vi "Dashboard Main.vi"() -> ()   [LabVIEW 2016]
uses:
  <vilib>/Utility/miscctls.llb/LVRowAndColumnTypeDef.ctl
  <vilib>/event_ctls.llb/eventvkey.ctl
  <vilib>/Rock Robotics/Network Tables/NT Read Numeric Array.vi
  <vilib>/Rock Robotics/Network Tables/NT Write Numeric Array.vi
  <vilib>/Rock Robotics/Network Tables/NT Write Boolean.vi
  <vilib>/Rock Robotics/WPI/Dashboard/WPI_DashboardLogging Global.vi
panel:
  in  "Camera Settings Right":T1={"Frame Rate"=30, "Compression"=30, "Size"=1, "DB Camera Config"=FALSE} {"Frame Rate" scale=1.0..30.0; "Compression" scale=100.0..-1.0; "Size" items=["640x480", "320x240", "160x120"]}
  in  "Camera Name Right":string(combo)="No Camera Selection"
  out "Camera Info":cluster{"Mbps LED":bool, "Mbps":dbl, "fps":dbl} {"fps" format="%#.1g"; "Mbps" format="%#.1g"}
  in  "Camera Settings":T1={"Frame Rate"=30, "Compression"=30, "Size"=1, "DB Camera Config"=FALSE} {"Frame Rate" scale=1.0..30.0; "Compression" scale=100.0..-1.0; "Size" items=["640x480", "320x240", "160x120"]}
  in  "TCP":refnum<k5>
  in  "Rec Mode":enum32{"Stop", "Record", "Playback"}(radio)
  out "Robot IP":string
  out "Image Message":string="Timeout in Camera Communications"
  in  "Dashboard Tab":T2(tab)
  in  "Robot Centric?":bool
  in  "Scooter Button":bool
  in  "Scooter Scale":dbl(slide)=0.49999999999999994 scale=0.0..1.0
  in  "Select Auto":string(combo)="Select Autonomous ..."
  out "NT Connection":bool
  out "MotorChart R":cluster{"Numeric":dbl, "Numeric":dbl}(graph)
  out "MotorChart L":cluster{"Numeric":dbl, "Numeric":dbl}(graph)
  out "MotorSliders R":cluster{"MotorSlide1":dbl, "MotorSlide2":dbl} {"MotorSlide2" scale=-1.0..1.0 scale format="%#_2e"; "MotorSlide1" scale=-1.0..1.0 scale format="%#_2e"}
  out "MotorSliders L":cluster{"MotorSlide1":dbl, "MotorSlide2":dbl} {"MotorSlide2" scale=-1.0..1.0 scale format="%#_2e"; "MotorSlide1" scale=-1.0..1.0 scale format="%#_2e"}
  out "Gyro":dbl(knob) scale=0.0..360.0
  out "JS1 Z":dbl(slide) scale=-1.0..1.0 scale format="%#_2e"
  out "JS1 Graph":cluster{"X":dbl, "Y":dbl}[](graph)
  out "JS1 Buttons":T3
  out "JS2 Z":dbl(slide) scale=-1.0..1.0 scale format="%#_2e"
  out "JS2 Graph":cluster{"X":dbl, "Y":dbl}[](graph)
  out "JS2 Buttons":T3
  out "Mode":T4(ring)=enum."Auto Disabled"
  out "Camera Image Right":T5(plugin-control)
  in  "DB/String 9":string
  in  "DB/String 8":string
  in  "DB/String 7":string
  in  "DB/String 6":string
  in  "DB/String 5":string
  in  "DB/String 4":string
  in  "DB/String 3":string
  in  "DB/String 2":string
  in  "DB/String 1":string
  in  "DB/String 0":string
  in  "DB/Slider 0":dbl(slide) scale=0.0..5.0
  in  "DB/Slider 1":dbl(slide) scale=0.0..5.0
  in  "DB/Slider 2":dbl(slide) scale=0.0..5.0
  in  "DB/Slider 3":dbl(slide) scale=0.0..5.0
  out "DB/LED 3":bool
  out "DB/LED 2":bool
  out "DB/LED 1":bool
  out "DB/LED 0":bool
  in  "DB/Button 3":bool
  in  "DB/Button 2":bool
  in  "DB/Button 1":bool
  in  "DB/Button 0":bool caption="New Name"
  out "Ultrasonic Distance":dbl
  out "Motor Outputs":T6 {"Motor 7" scale=-1.0..1.0; "Motor 6" scale=-1.0..1.0; "Motor 5" scale=-1.0..1.0; "Motor 4" scale=-1.0..1.0; "Motor 3" scale=-1.0..1.0; "Motor 2" scale=-1.0..1.0; "Motor 1" scale=-1.0..1.0; "Motor 0" scale=-1.0..1.0}
  in  "PID Adjustments":cluster{"P":dbl, "I":dbl, "D":dbl}={"P"=0.3, "I"=0.0, "D"=0.004} {"D" min=0.0 max=10.0 step=0.01; "I" min=0.0 max=10.0 step=0.01; "P" min=0.0 max=10.0 step=0.01}
  out "Encoder Data":dbl[](array[numeric])
  out "NavX Data":dbl[](array[numeric])
  in  "Encoder Offsets":dbl[](array[numeric])
  in  "Test Slider":dbl(slide) scale=0.0..100.0 scale format="%#_3g"
  in  "On/Off":bool caption="Solenoid"
  in  "Test Name":u16(ring) items=["Select the test to run..."]
  in  "Test Tree":string(tree)
  in  "Motor":cluster{"Value":dbl, "Enable":bool} {"Value" scale=-1.0..1.0 scale format="%#_3g"}
  out "Progress":T7 {"Test Progress" scale=0.0..100.0}
  in  "Rev/Fwd":cluster{"Forward":bool, "Reverse":bool}
  in  "Test Ring":u16(ring) items=["Monochrome", "Color"]
  out "Cmd Status":string
  in  "Execute Command":bool
  in  "Command Params":string[][](table)
  in  "Command Selection":i32(listbox)
  in  "CheckList":i32(listbox)
  out "Tree":string(tree)
  out "30 Amp Plugs":dbl[](array[slide]) scale=0.0..30.0
  out "40 Amp Plugs":dbl[](array[slide]) scale=0.0..40.0
  out "Camera Image":T5(plugin-control)
  out "Background":bool
  in  "Camera Name":string(combo)="No Camera Selection"
  # "HW"
  # "HW"
  # "Joysticks"
  # "Drive Motors"
  # "Front"
  # "Right"
  # "Left"
  # "Back"
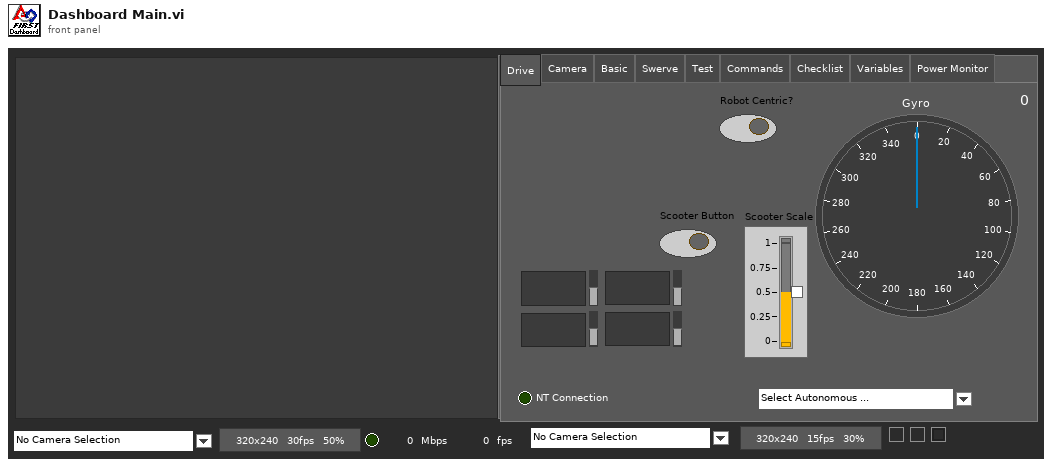
[diagram p1: front panel]
types:
  T1 = cluster{"Frame Rate":i32, "Compression":i32, "Size":u16, "DB Camera Config":bool}
  T2 = enum32{"Drive", "Camera", "Basic", "Swerve", "Test", "Commands", "Checklist", "Variables", "Power Monitor"}
  T3 = cluster{bool, bool, bool, bool, bool, bool, bool, bool, bool, bool, bool, bool}
  T4 = enum8{"Tele-Op Disabled", "Tele-Op Enabled", "Auto Disabled", "Auto Enabled", "Test Disabled", "Test Enabled", "Disconnected", "No Code", "E-Stop"}
  T5 = typedef "IMAQ Image.ctl" = refnum<image>
  T6 = cluster{"Motor 0":dbl, "Motor 1":dbl, "Motor 2":dbl, "Motor 3":dbl, "Motor 4":dbl, "Motor 5":dbl, "Motor 6":dbl, "Motor 7":dbl}
  T7 = cluster{"Test Progress":u8, "Test Progress Text":string}
  T8 = typedef "Image Type" = u32
  T9 = cluster{"IDs":cluster{"RPC field ID":u16, "Unique ID":u16}, "String":string}
  T10 = enum32{"Drive", "Basic", "Custom", "Test", "Checklist", "Variables"}
  T11 = cluster{"Error Strings":string, "Disable Counts":cluster{u16, u16}, "Rail Faults":cluster{u16, u16, u16}, "Robot IP":string, "DB Mode":u8, "Event Info":cluster{"Name":string, "Type":u8, "Number":u16, "Replay":u8}}
  T12 = cluster{"Storage":cluster{"Disk Free":u64, "RAM Block":u32, "RAM free":u32}, "CPU Utilization":cluster{"CPU % ISR":sgl, "CPU % Time Crit":sgl, "CPU % Timed Str":sgl, "CPU % High":sgl, "CPU % Above":sgl, "CPU % Normal":sgl, "CPU % Low":sgl}, "CAN":cluster{"% Bus Utilization":sgl, "Bus Off Cnt":u32, "TX_FIFO Full Cnt":u32, "Receive Error Cnt":u8, "Transmit Error Cnt":u8}, "HID":cluster{"HID Outputs":u32, "Rumble Low":u16, "Rumble High":u16}[]}
  T13 = cluster{"Status bits":cluster{"Test Mode":bool, "Autonomous":bool, "Enabled":bool, "Code Start":bool, "Brownout":bool, "Reserved 2":bool, "Reserved 3":bool, "E-Stop":bool}, "Code Trace":cluster{"Disabled":bool, "TeleOp":bool, "Auto":bool, "Test":bool}, "Controller Type":enum16{"unknown", "cRIO", "roboRio"}, "Code?":enum16{"unknown", "noCode", "code"}, "Battery V":dbl}
  T14 = cluster{"Control Bits":cluster{"TestMode":bool, "Autonomous":bool, "Enabled":bool, "FMS Present":bool, bool, bool, bool, "E-Stop":bool}, "Team Station ":u8, "Countdown":sgl, "Joystick Values":cluster{"Axes":dbl[], "Buttons":bool[], "POVs":i16[]}[]}
  T15 = cluster{"Axes":dbl[], "Buttons":bool[], "POVs":i16[]}[]
  T16 = cluster{"Numeric Array[0]":dbl, "Numeric Array[1]":dbl, "Numeric Array[2]":dbl, "Numeric Array[3]":dbl, "Numeric Array[4]":dbl, "Numeric Array[5]":dbl, "Numeric Array[6]":dbl, "Numeric Array[7]":dbl, "Numeric Array[8]":dbl}
  T17 = cluster{"Numeric Array[0]":dbl, "Numeric Array[1]":dbl, "Numeric Array[2]":dbl, "Numeric Array[3]":dbl, "Numeric Array[4]":dbl, "Numeric Array[5]":dbl, "Numeric Array[6]":dbl, "Numeric Array[7]":dbl}
  T18 = cluster{"Axes":dbl[], "Buttons":bool[], "POVs":i16[]}
  T19 = cluster{"Buttons[0]":bool, "Buttons[1]":bool, "Buttons[2]":bool, "Buttons[3]":bool, "Buttons[4]":bool, "Buttons[5]":bool, "Buttons[6]":bool, "Buttons[7]":bool, "Buttons[8]":bool, "Buttons[9]":bool, "Buttons[10]":bool, "Buttons[11]":bool}
  T20 = cluster{"Camera Image":refnum<vi>, "Dashboard Tab":refnum<vi>, "Background":refnum<vi>, "Rec Mode":refnum<vi>, "Test Slider":refnum<vi>, "On/Off ":refnum<vi>, "Test Ring":refnum<vi>, "Rev/Fwd":refnum<vi>, "Test Name":refnum<vi>, "Motor":refnum<vi>, "Progress":refnum<vi>, "CheckList":refnum<vi>, "Tree":refnum<vi>, "Test Tree":refnum<vi>, "Command Params":refnum<vi>, "Command Selection":refnum<vi>, "Execute Command":refnum<vi>, "Cmd Status":refnum<vi>, "Camera Settings":refnum<vi>, "Camera Name":refnum<vi>, "Camera Info":refnum<vi>, "Camera Settings Right":refnum<vi>, "Camera Name Right":refnum<vi>, "Camera Image Right":refnum<vi>}
  T21 = cluster{"Operation":enum16{"Update", "Clear"}, "Color Box":u32}[]
  T22 = typedef "eventvkey.ctl" = enum16{"ASCII", "Enter", "Return", "Shift", "Ctrl", "Alt", "Cmd", "Opt", "Caps", "NumLock", "Clear", "Break", "Up", "Down", "Left", "Right", "Insert", "Delete", "Home", "End", "PageUp", "PageDown", "Escape", "Help", "Pause", "ScrollLock", "F1", "F2", "F3", "F4", "F5", "F6", "F7", "F8", "F9", "F10", "F11", "F12", "F13", "F14", "F15", "F16", "F17", "F18", "F19", "F20", "F21", "F22", "F23", "F24", "Play", "VolumeUp", "VolumeDown", "Mute", "Two Byte Char"}
  T23 = cluster{"Image Size":bool, "Image Type":bool, "Pixel Value":bool, "ROI Information":bool, "Zoom Factor":bool}
  T24 = cluster{"Operation":enum16{"Update", "Clear"}, "Color Box":u32}
  T25 = typedef "LVRowAndColumnTypeDef.ctl" = cluster{"Row":i32, "Column":i32}
  T26 = cluster{"Shift":bool, "Ctrl":bool, "Alt":bool, "Cmd":bool, "Opt":bool}
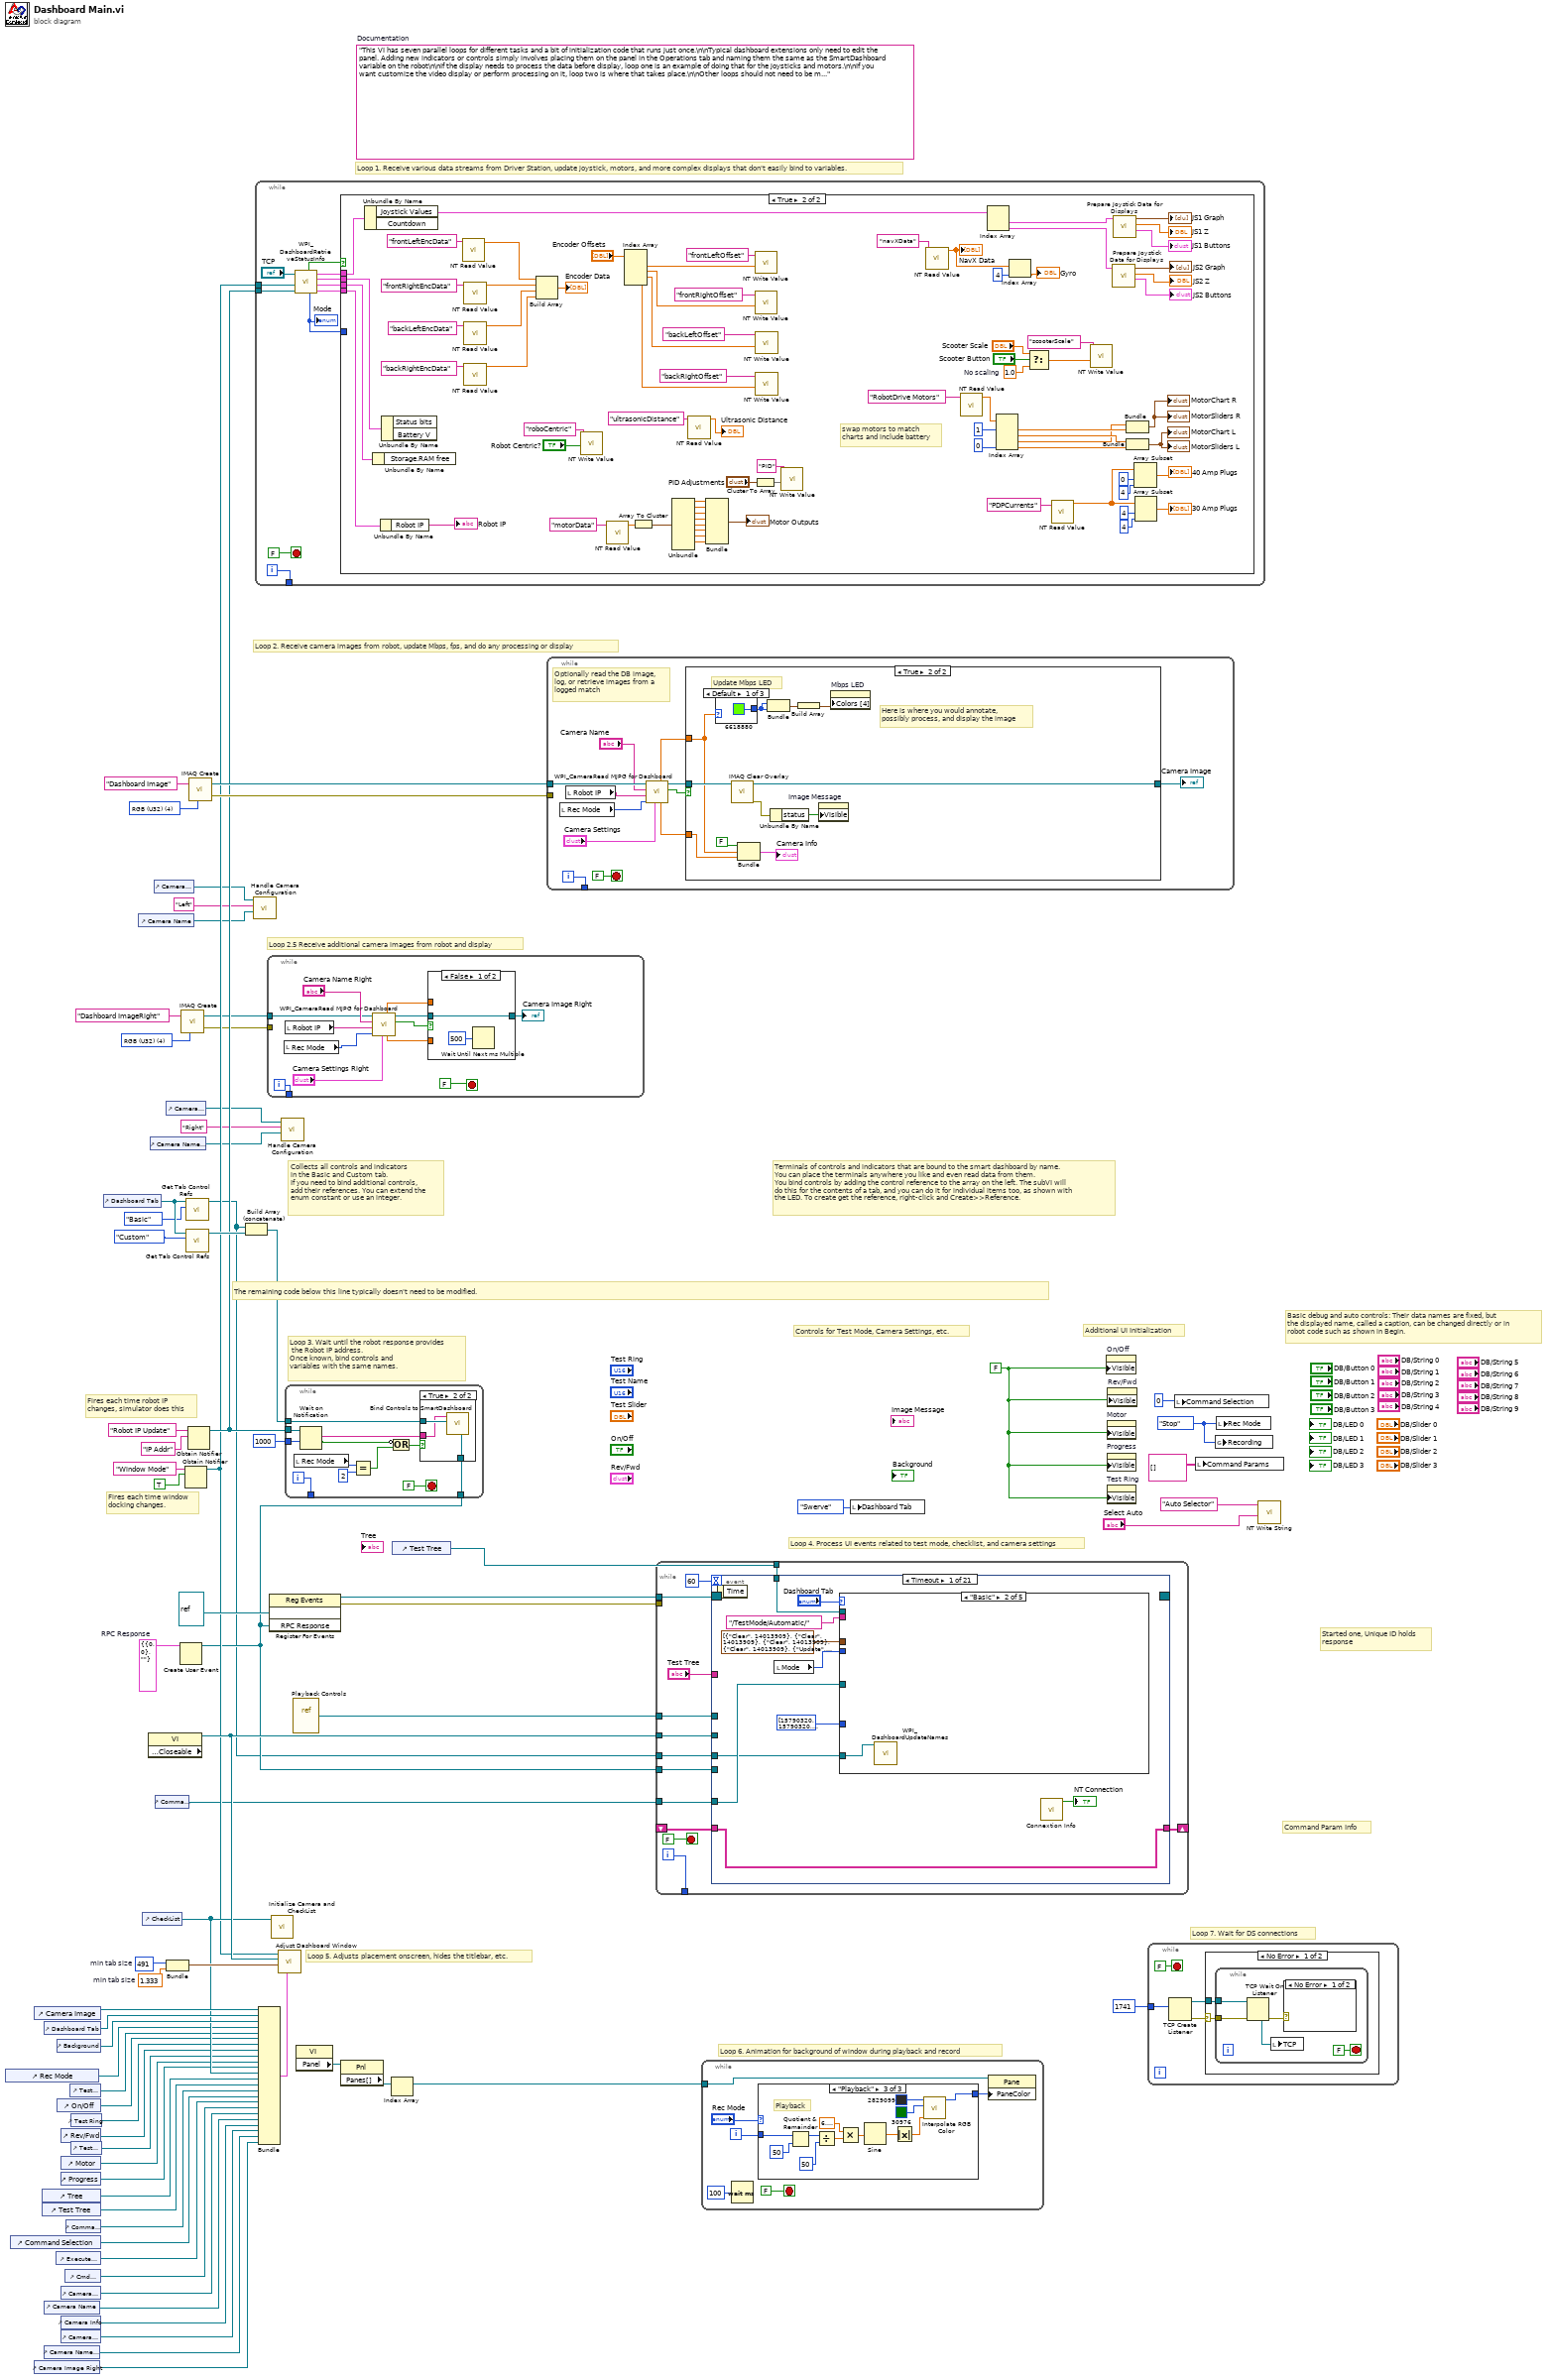
[diagram p0: block diagram]
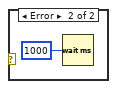
[diagram p3: hidden frame]
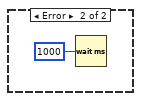
[diagram p4: hidden frame]
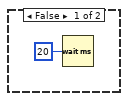
[diagram p5: hidden frame]
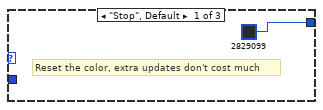
[diagram p6: hidden frame]
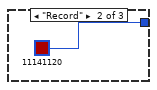
[diagram p7: hidden frame]
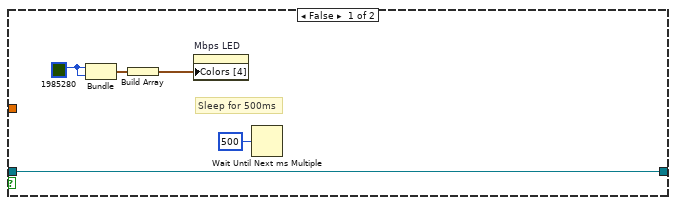
[diagram p9: hidden frame]
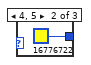
[diagram p10: hidden frame]
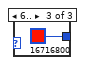
[diagram p11: hidden frame]
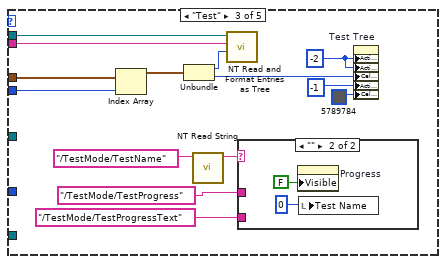
[diagram p13: hidden frame]
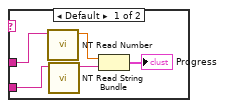
[diagram p14: hidden frame]
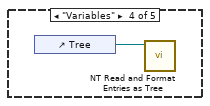
[diagram p15: hidden frame]
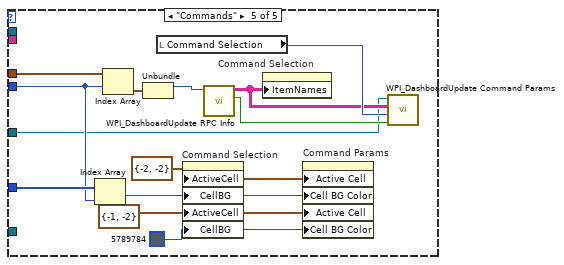
[diagram p16: hidden frame]
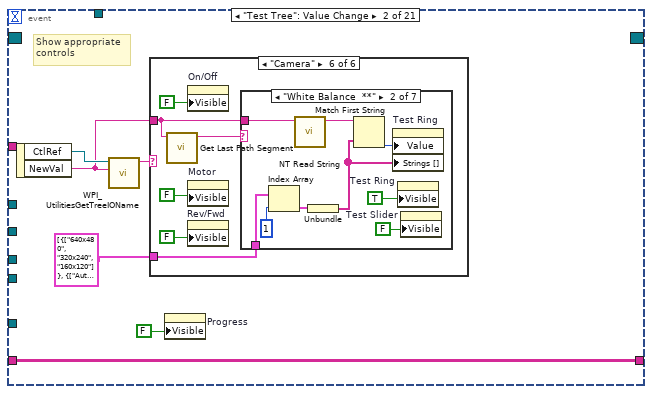
[diagram p17: hidden frame]
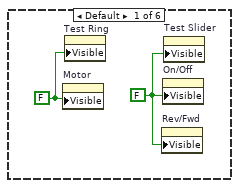
[diagram p18: hidden frame]
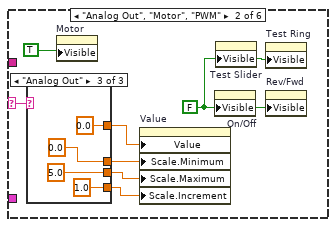
[diagram p19: hidden frame]
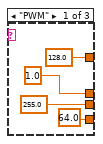
[diagram p20: hidden frame]
diagram:
  w11 = T8 4 items=["Grayscale (U8)", "Grayscale (I16)", "Grayscale (SGL)", "Complex (CSG)", "RGB (U32)", "HSL (U32)", "RGB (U64)"] ("Image Type")
  w27 = T9 {"IDs"={"RPC field ID"=0, "Unique ID"=0}, "String"=""}  # RPC Response
  w51 = 491  # min tab size
  w50 = 1.333  # min tab size
  w58 = enum32{"Stop", "Record", "Playback"}."Stop" ("Rec Mode")
  w33 = FALSE ("Visible")
  (unwired) "This VI has seven parallel loops for different tasks and a bit of initialization code that runs just once.\n\nTypical dashboard extensions only need to edit the panel. Adding new indicators or controls simply involves placing them on the panel in the Operations tab and naming them the same as the SmartDashboard variable on the robot\n\nIf the display needs to process the data before display, loop one is an example of doing that for the joysticks and motors.\n\nIf you want customize the video display or perform processing on it, loop two is where that takes place.\n\nOther loops should not need to be modified. They are pretty standard, and document the task they perform."  # Documentation
  w75 = T8 4 items=["Grayscale (U8)", "Grayscale (I16)", "Grayscale (SGL)", "Complex (CSG)", "RGB (U32)", "HSL (U32)", "RGB (U64)"] ("Image Type")
  # "Loop 2.5 Receive additional camera images from robot and display"
  # "Command Param Info"
  # "Started one, Unique ID holds\nresponse"
  # "Loop 7. Wait for DS connections"
  # "Basic debug and auto controls: Their data names are fixed, but\nthe displayed name, called a caption, can be changed directly or in\nrobot code such as shown in Begin."
  # "Controls for Test Mode, Camera Settings, etc."
  # "Additional UI Initialization"
  # "Loop 6. Animation for background of window during playback and record"
  # "Fires each time robot IP\nchanges, simulator does this"
  # "Fires each time window\ndocking changes."
  # "Collects all controls and indicators\nin the Basic and Custom tab.\nIf you need to bind additional controls,\nadd their references. You can extend the\nenum constant or use an integer."
  # "The remaining code below this line typically doesn't need to be modified."
  # "Loop 4. Process UI events related to test mode, checklist, and camera settings"
  # "Terminals of controls and indicators that are bound to the smart dashboard by name.\nYou can place the terminals anywhere you like and even read data from them.\nYou bind controls by adding the control reference to the array on the left. The subVI will\ndo this for the contents of a tab, and you can do it for individual items too, as shown with\nthe LED. To create get the reference, right-click and Create>>Reference."
  # "Loop 3. Wait until the robot response provides\n the Robot IP address.\nOnce known, bind controls and\nvariables with the same names."
  # "Loop 5. Adjusts placement onscreen, hides the titlebar, etc."
  # "Loop 1. Receive various data streams from Driver Station, update joystick, motors, and more complex displays that don't easily bind to variables."
  # "Loop 2. Receive camera images from robot, update Mbps, fps, and do any processing or display"
  n1 = control-ref of="Rec Mode"() -> (w39:refnum<vi>)
  n2 = control-ref of="Command Selection"() -> (w26:refnum<vi>)
  n3 = control-ref of="Camera Image Right"() -> (w2:refnum<vi>)
  n4 = control-ref of="Camera Image"() -> (w53:refnum<vi>)
  n5 = control-ref of="Tree"() -> (w43:refnum<vi>)
  n6 = control-ref of="Test Tree"() -> (w42:refnum<vi>)
  n7 = control-ref of="Dashboard Tab"() -> (w52:refnum<vi>)
  n8 = control-ref of="Camera Name"() -> (w17:refnum<vi>)
  n9 = control-ref of="Camera Name Right"() -> (w3:refnum<vi>)
  n10 = control-ref of="Execute Command"() -> (w28:refnum<vi>)
  n11 = control-ref of="Background"() -> (w48:refnum<vi>)
  n12 = control-ref of="On/Off"() -> (w37:refnum<vi>)
  n13 = control-ref of="Progress"() -> (w34:refnum<vi>)
  n14 = control-ref of="Camera Settings"() -> (w18:refnum<vi>)
  n15 = control-ref of="Camera Info"() -> (w16:refnum<vi>)
  n16 = control-ref of="Camera Settings Right"() -> (w4:refnum<vi>)
  n17 = control-ref of="Rev/Fwd"() -> (w35:refnum<vi>)
  n18 = control-ref of="Motor"() -> (w40:refnum<vi>)
  n19 = control-ref of="Cmd Status"() -> (w22:refnum<vi>)
  n20 = control-ref of="Command Params"() -> (w29:refnum<vi>)
  n21 = control-ref of="Test Slider"() -> (w38:refnum<vi>)
  n22 = control-ref of="Test Ring"() -> (w36:refnum<vi>)
  n23 = control-ref of="Test Name"() -> (w41:refnum<vi>)
  n24 = control-ref of="Dashboard Tab"() -> (w56:refnum<vi>)
  n25 = control-ref of="Camera Name"() -> (w19:refnum<vi>)
  n26 = control-ref of="CheckList"() -> (w44:refnum<vi>)
  n27 = property class="VI" props=["Front Panel.Closeable"]() -> (reference out=w57:refnum<vi>)  [unwired: 2 in, 2 out]
  n28 = control-ref of="Camera Name Right"() -> (w7:refnum<vi>)
  n29 = control-ref of="Camera Settings"() -> (w20:refnum<vi>)
  n30 = control-ref of="Command Params"() -> (w21:refnum<vi>)
  n31 = control-ref of="Camera Settings Right"() -> (w8:refnum<vi>)
  n32 = Bundle("min tab size"=w51, "min tab size"=w50) -> (w49:cluster{"min tab size":i32, "min tab size":dbl})  [unwired: 1 in]
  n33 = Create User Event(user event datatype=w27) -> (user event=w23:refnum<user-event>)  [unwired: 1 in, 1 out]
  n34 = call "IMAQ Create"("Image Name"="Dashboard ImageRight", "Image Type"=w11) -> ("New Image"=w10:T5, "error out"=w9:errorcluster)  [unwired: 2 in, 1 out]
  n35 = Obtain Notifier(name (unnamed)="Window Mode", notification data type=TRUE) -> (notifier out=w31:refnum<notifier>)  [unwired: 2 in, 2 out]
  n36 = call <vilib>:"Get Tab Control Refs.vi"("Page Index"=T10."Basic" ("Dashboard Tab"), "TabControl in"=w56) -> ("ControlsOnPage"=w15:refnum<vi>[])  [unwired: 9 in]
  n37 = call <vilib>:"Get Tab Control Refs.vi"("Page Index"=T10."Custom" ("Dashboard Tab"), "TabControl in"=w56) -> ("ControlsOnPage"=w55:refnum<vi>[])  [unwired: 9 in]
  n38 = Obtain Notifier(name (unnamed)="Robot IP Update", notification data type="IP Addr" ("name (unnamed)")) -> (notifier out=w32:refnum<notifier>)  [unwired: 2 in, 2 out]
  n39 = call "IMAQ Create"("Image Name"="Dashboard Image", "Image Type"=w75) -> ("New Image"=w73:T5, "error out"=w72:errorcluster)  [unwired: 2 in, 1 out]
  n40 = Build Array (concatenate)(w15, w55) -> (w54:refnum<vi>[])
  n41 = call "Handle Camera Configuration.vi"("CameraNameRef"=w19, "Camera File Name"="Left", "ClusterRef"=w20) -> ()  [unwired: 9 in]
  n42 = while {
    tunnel: [w85] -> _
    tunnel: w32 -> [w79]
    tunnel: w31 -> [w76]
    i -> [w85]
    stop <- FALSE stop-if-true
    n43 = call <vilib>:"WPI_DashboardRetrieveStatusInfo.vi"("Binding Refnum"=w79, "Window Mode Notifier"=w76, "TCP Cnx"="TCP") -> ("Power and Errors"=w80:T11, "Robot Metrics"=w83:T12, "Status Info"=w84:T13, "Control Info"=w81:T14, "Robot Mode"=w78:T4, "Process?"=w82:bool)  [unwired: 3 in]
    "Mode" <- w78
    n44 = case shown="True" w82 {
      tunnel: w84 -> [_ w165]
      tunnel: w83 -> [_ w164]
      tunnel: w81 -> [_ w163]
      tunnel: w80 -> [_ w162]
      tunnel: w78 -> [_ _]
      frame False {
        n45 = Wait (ms)(milliseconds to wait=u32 20) -> ()  [unwired: 1 out]
      }
      frame True {
        w94 = 1.0  # No scaling
        # "swap motors to match\ncharts and include battery"
        n46 = Unbundle By Name(w163) -> ("Joystick Values"=w153:T15)  [unwired: 1 out]
        n47 = Unbundle By Name(w164) -> ()  [unwired: 1 out]
        n48 = Unbundle By Name(w162) -> ("Robot IP"=→"Robot IP":string)
        n49 = Unbundle By Name(w165) -> ()  [unwired: 2 out]
        n50 = call-poly <vilib>:"NT Read Value.vi"("Name"="frontLeftEncData") -> ("Numeric"=w127:dbl)  [unwired: 9 in, 1 out]
        n51 = call-poly <vilib>:"NT Read Value.vi"("Name"="frontRightEncData") -> ("Numeric"=w126:dbl)  [unwired: 9 in, 1 out]
        n52 = call-poly <vilib>:"NT Read Value.vi"("Name"="backLeftEncData") -> ("Numeric"=w125:dbl)  [unwired: 9 in, 1 out]
        n53 = call-poly <vilib>:"NT Read Value.vi"("Name"="backRightEncData") -> ("Numeric"=w124:dbl)  [unwired: 9 in, 1 out]
        n54 = Build Array(w127, w126, w125, w124) -> (→"Encoder Data":dbl[])
        n55 = call-poly <vilib>:"NT Write Value.vi"("Boolean"="Robot Centric?", "Name"="roboCentric") -> ()  [unwired: 9 in, 1 out]
        n56 = call-poly <vilib>:"NT Read Value.vi"("Name"="motorData") -> ("Numeric Array"=w118:dbl[])  [unwired: 9 in, 1 out]
        n57 = Index Array(array="Encoder Offsets") -> (element #1=w135:dbl, element #2=w134:dbl, element #3=w133:dbl, element #4=w132:dbl)  [unwired: 4 in]
        n58 = Array To Cluster(array=w118) -> (cluster=w117:T16)
        n59 = Unbundle(w117) -> ("Numeric Array[0]"=w116:dbl, "Numeric Array[1]"=w115:dbl, "Numeric Array[2]"=w114:dbl, "Numeric Array[3]"=w113:dbl, "Numeric Array[4]"=w112:dbl, "Numeric Array[5]"=w111:dbl, "Numeric Array[6]"=w110:dbl, "Numeric Array[7]"=w109:dbl)  [unwired: 1 out]
        n60 = call-poly <vilib>:"NT Read Value.vi"("Name"="ultrasonicDistance") -> ("Numeric"=→"Ultrasonic Distance":dbl)  [unwired: 9 in, 1 out]
        n61 = Bundle("Numeric Array[0]"=w116, "Numeric Array[1]"=w115, "Numeric Array[2]"=w114, "Numeric Array[3]"=w113, "Numeric Array[4]"=w112, "Numeric Array[5]"=w111, "Numeric Array[6]"=w110, "Numeric Array[7]"=w109) -> (→"Motor Outputs":T17)  [unwired: 1 in]
        n62 = Cluster To Array(cluster="PID Adjustments") -> (array=w121:dbl[])
        n63 = call-poly <vilib>:"NT Write Value.vi"("Numeric"=w135, "Name"="frontLeftOffset") -> ()  [unwired: 9 in, 1 out]
        n64 = call-poly <vilib>:"NT Write Value.vi"("Numeric"=w134, "Name"="frontRightOffset") -> ()  [unwired: 9 in, 1 out]
        n65 = call-poly <vilib>:"NT Write Value.vi"("Numeric"=w133, "Name"="backLeftOffset") -> ()  [unwired: 9 in, 1 out]
        n66 = call-poly <vilib>:"NT Write Value.vi"("Numeric"=w132, "Name"="backRightOffset") -> ()  [unwired: 9 in, 1 out]
        n67 = call-poly <vilib>:"NT Write Value.vi"("Numeric Array"=w121, "Name"="PID") -> ()  [unwired: 9 in, 1 out]
        n68 = call-poly <vilib>:"NT Read Value.vi"("Name"="navXData") -> ("Numeric Array"=w107:dbl[])  [unwired: 9 in, 1 out]
        "NavX Data" <- w107
        n69 = call-poly <vilib>:"NT Read Value.vi"("Name"="RobotDrive Motors") -> ("Numeric Array"=w143:dbl[])  [unwired: 9 in, 1 out]
        n70 = Index Array(array=w153) -> (element #1=w152:T18, element #2=w148:T18)  [unwired: 2 in]
        n71 = Index Array(array=w143, index #1=1, index #4=0) -> (element #1=w157:dbl, element #2=w158:dbl, element #3=w156:dbl, element #4=w161:dbl)  [unwired: 2 in]
        n72 = Index Array(array=w107, index=4) -> (element=→"Gyro":dbl)
        n73 = Select(t="Scooter Scale", s="Scooter Button", f=w94) -> (s? t:f=w93:dbl)
        n74 = call-poly <vilib>:"NT Read Value.vi"("Name"="PDPCurrents") -> ("Numeric Array"=w101:dbl[])  [unwired: 9 in, 1 out]
        n75 = call-poly <vilib>:"NT Write Value.vi"("Numeric"=w93, "Name"="scooterScale") -> ()  [unwired: 9 in, 1 out]
        n76 = call "Prepare Joystick Data for Displays.vi"("Joystick Values"=w148) -> ("Buttons"=→"JS2 Buttons":T19, "Z Axis"=→"JS2 Z":dbl, "Cartesian Data"=→"JS2 Graph":cluster{"X axis":dbl, "X axis":dbl}[])  [unwired: 8 in]
        n77 = call "Prepare Joystick Data for Displays.vi"("Joystick Values"=w152) -> ("Buttons"=→"JS1 Buttons":T19, "Z Axis"=→"JS1 Z":dbl, "Cartesian Data"=→"JS1 Graph":cluster{"X axis":dbl, "X axis":dbl}[])  [unwired: 8 in]
        n78 = Bundle("Numeric"=w156, "Numeric"=w157) -> (→"MotorChart R" →"MotorSliders R":cluster{"Numeric":dbl, "Numeric":dbl})  [unwired: 1 in]
        n79 = Bundle("Numeric"=w158, "Numeric"=w161) -> (→"MotorChart L" →"MotorSliders L":cluster{"Numeric":dbl, "Numeric":dbl})  [unwired: 1 in]
        n80 = Array Subset(array=w101, index=0, length=4) -> (→"40 Amp Plugs":dbl[])
        n81 = Array Subset(array=w101, index=4, length=4) -> (→"30 Amp Plugs":dbl[])
      }
    }
  }
  n82 = Bundle("Camera Image"=w53, "Dashboard Tab"=w52, "Background"=w48, "Rec Mode"=w39, "Test Slider"=w38, "On/Off"=w37, "Test Ring"=w36, "Rev/Fwd"=w35, "Test Name"=w41, "Motor"=w40, "Progress"=w34, "CheckList"=w44, "Tree"=w43, "Test Tree"=w42, "Command Params"=w29, "Command Selection"=w26, "Execute Command"=w28, "Cmd Status"=w22, "Camera Settings"=w18, "Camera Name"=w17, "Camera Info"=w16, "Camera Settings Right"=w4, "Camera Name Right"=w3, "Camera Image Right"=w2) -> (w45:T20)  [unwired: 1 in]
  n83 = while {
    tunnel: w10 -> [w176]
    tunnel: w9 -> [_]
    tunnel: [w170] -> _
    i -> [w170]
    stop <- FALSE stop-if-true
    n84 = local read "Rec Mode"() -> (w174:enum32{"Stop", "Record", "Playback"})
    n85 = local read "Robot IP"() -> (w175:string)
    n86 = call <vilib>:"WPI_CameraRead MJPG for Dashboard.vi"("Camera Settings"="Camera Settings Right", "Rec Mode"=w174, "Robot IP"=w175, "Camera Name"="Camera Name Right", "Refnum in"=w176) -> ("Active"=w169:bool, "Refnum out"=w172:T5, "FPS"=w167:dbl, "Bandwidth (Mbps)"=w168:dbl)  [unwired: 3 in]
    n87 = case shown="False" w169 {
      tunnel: w172 -> [w178 w180]
      tunnel: w168 -> [_ _]
      tunnel: w167 -> [_ _]
      tunnel: [w178 w180] -> w166
      frame False {
        n88 = Wait Until Next ms Multiple(millisecond multiple=u32 500) -> ()  [unwired: 1 out]
      }
      frame True {
      }
    }
    "Camera Image Right" <- w166
  }
  n89 = register-events(refnum<vi> refnum, w23) -> (reference out=w62:refnum<event-registration>, error out=w61:errorcluster)  [unwired: 2 in]
  n90 = call "Initialize Camera and CheckList.vi"("ListBox in"=w44) -> ()  [unwired: 11 in]
  n91 = call "Adjust Dashboard Window.vi"("Sizing Refnums"=w45, "Size Constraints"=w49, "VI"=w57, "WIn Mode"=w31) -> ()  [unwired: 8 in]
  n92 = call "Handle Camera Configuration.vi"("CameraNameRef"=w7, "Camera File Name"="Right", "ClusterRef"=w8) -> ()  [unwired: 9 in]
  n93 = while {
    tunnel: w54 -> [w192]
    tunnel: w32 -> [w190]
    tunnel: [w188] -> _
    tunnel: u32 1000 ("milliseconds to wait") -> [w187]
    tunnel: w23 -> [w181]
    i -> [w188]
    stop <- FALSE stop-if-true
    n94 = local read "Rec Mode"() -> (w183:enum32{"Stop", "Record", "Playback"})
    n95 = Wait on Notification(notifier=w190, timeout in ms (-1)=w187) -> (notification=w189:string, timed out?=w185:bool)  [unwired: 2 in, 2 out]
    n96 = Equal?(x=w183, y=u16 2 ("Rec Mode")) -> (x = y?=w184:bool)
    n97 = Compound Arithmetic op=OR(invert w185, w184) -> (w186:bool)
    n98 = case shown="True" w186 {
      tunnel: w192 -> [_ w195]
      tunnel: w189 -> [_ w194]
      tunnel: w181 -> [_ w193]
      frame False {
      }
      frame True {
        n99 = call <vilib>:"Bind Controls to SmartDashboard.vi"("RPC ref"=w193, "Bound Control Refs"=w195, "Server IP Address"=w194) -> ()  [unwired: 9 in]
      }
    }
  }
  n100 = vi-ref "Playback Controls.vi"() -> (w63:refnum<vi>)
  n101 = property class="VI"() -> ("Panel"=w65:refnum<vi>)  [unwired: 2 in, 2 out]
  n102 = property class="Pnl"(reference=w65) -> ("Panes[]"=w66:refnum<vi>[])  [unwired: 1 in, 2 out]
  n103 = Index Array(array=w66) -> (element=w64:refnum<vi>)  [unwired: 1 in]
  n104 = control-ref of="Test Tree"() -> (w67:refnum<vi>)
  n105 = while {
    tunnel: w73 -> [w205]
    tunnel: w72 -> [_]
    tunnel: [w206] -> _
    i -> [w206]
    stop <- FALSE stop-if-true
    # "Optionally read the DB image,\nlog, or retrieve images from a\nlogged match"
    n106 = local read "Rec Mode"() -> (w201:enum32{"Stop", "Record", "Playback"})
    n107 = local read "Robot IP"() -> (w200:string)
    n108 = call <vilib>:"WPI_CameraRead MJPG for Dashboard.vi"("Camera Settings"="Camera Settings", "Rec Mode"=w201, "Robot IP"=w200, "Camera Name"="Camera Name", "Refnum in"=w205) -> ("Active"=w203:bool, "Refnum out"=w204:T5, "FPS"=w202:dbl, "Bandwidth (Mbps)"=w199:dbl)  [unwired: 3 in]
    n109 = case shown="True" w203 {
      tunnel: w204 -> [w208 w219]
      tunnel: w199 -> [_ w216]
      tunnel: w202 -> [_ w217]
      tunnel: [w208 w213] -> w196
      frame False {
        w210 = u32 1985280 ("Color Box")
        # "Sleep for 500ms"
        n110 = Bundle("Color Box"=w210, "Color Box"=w210) -> (w211:cluster{"Color Box":u32, "Color Box":u32})  [unwired: 1 out]
        n111 = Build Array(w211) -> (w209:cluster{"Color Box":u32, "Color Box":u32}[])
        n112 = property on="Mbps LED" class="Bool (strict)"("Colors [4]"=w209) -> ()  [unwired: 2 in, 2 out]
        n113 = Wait Until Next ms Multiple(millisecond multiple=u32 500) -> ()  [unwired: 1 out]
      }
      frame True {
        # "Here is where you would annotate,\npossibly process, and display the image"
        # "Update Mbps LED"
        n114 = case shown="Default" w216 {
          tunnel: [u32 6618880 ("Color Box") u32 16776722 ("Color Box") u32 16716800 ("Color Box")] -> w220
          frame Default {
          }
          frame 4, 5 {
          }
          frame 6.. {
          }
        }
        n115 = call "IMAQ Clear Overlay"("Image"=w219) -> ("error out"=w222:errorcluster, "Image Out"=w213:T5)  [unwired: 2 in, 7 out]
        n116 = Bundle(FALSE, "Bandwidth (Mbps)"=w216, "FPS"=w217) -> (→"Camera Info":cluster{bool, "Bandwidth (Mbps)":dbl, "FPS":dbl})  [unwired: 1 in]
        n117 = Bundle("Color Box"=w220, "Color Box"=w220) -> (w221:cluster{"Color Box":u32, "Color Box":u32})  [unwired: 1 out]
        n118 = Unbundle By Name(w222) -> ("status"=w223:bool)
        n119 = Build Array(w221) -> (w218:cluster{"Color Box":u32, "Color Box":u32}[])
        n120 = property on="Image Message" class="Str"("Visible"=w223) -> ()  [unwired: 2 in, 2 out]
        n121 = property on="Mbps LED" class="Bool (strict)"("Colors [4]"=w218) -> ()  [unwired: 2 in, 2 out]
      }
    }
    "Camera Image" <- w196
  }
  n122 = while {
    tunnel: [w236] -> _
    tunnel: w67 -> [w235]
    tunnel: w63 -> [w234]
    tunnel: w62 -> [w233]
    tunnel: w61 -> [_]
    tunnel: w57 -> [w232]
    tunnel: w23 -> [w231]
    tunnel: w21 -> [w230]
    shift-right: [w229] -> _
    shift-left: _ -> [w228]
    tunnel: w15 -> [w227]
    i -> [w236]
    stop <- FALSE stop-if-true
    n123 = event shown="[0] Timeout" {
      selector: w233 -> [_ _ _ _ _ _ _ _ _ _ _ _ _ _ _ _ _ _ _ _ _]
      dyn-events: [_ _ _ _ _ _ _ _ _ _ _ _ _ _ _ _ w492 _ _ _ _] -> _
      timeout: u32 60 ("milliseconds to wait") -> [_ _ _ _ _ _ _ _ _ _ _ _ _ _ _ _ _ _ _ _ _]
      tunnel: w235 -> [w248 _ _ _ _ _ _ _ _ _ _ _ _ _ _ _ _ _ _ _ _]
      tunnel: "Test Tree" -> [_ _ _ _ _ _ _ _ _ _ _ w459 w467 w469 w473 w481 _ _ _ _ _]
      tunnel: w234 -> [_ _ _ _ _ _ _ _ _ _ _ _ _ _ _ _ w494 _ w512 _ _]
      tunnel: w232 -> [_ _ _ _ _ _ _ _ _ _ _ _ _ _ _ _ w490 _ _ _ _]
      tunnel: w231 -> [_ _ _ _ _ _ _ _ _ _ _ _ _ _ _ _ w486 _ _ _ _]
      tunnel: w230 -> [w243 _ _ _ _ _ w410 _ _ _ _ _ _ _ _ _ _ _ _ _ _]
      tunnel: [w242 w287 w389 w394 w403 w407 w408 w417 w427 w434 w446 w458 w465 w468 w472 w480 w485 w507 w509 w513 w524] -> w229
      tunnel: w228 -> [w242 w287 w389 w394 w403 w407 w408 _ _ w434 w446 w458 w465 w468 w472 w480 w485 w507 w509 w513 w524]
      tunnel: w227 -> [w240 _ _ _ _ _ _ _ _ _ _ _ _ _ _ _ _ _ _ _ _]
      event Timeout {
        n124 = event-data() -> ()  [unwired: 1 in, 1 out]
        n125 = local read "Mode"() -> (w245:T4)
        n126 = case shown="\"Basic\"" "Dashboard Tab" {
          tunnel: w248 -> [_ _ w264 _ _]
          tunnel: "/TestMode/Automatic/" ("Name Pattern") -> [_ _ w263 _ _]
          tunnel: T21 [{"Operation"=enum."Clear", "Color Box"=14013909}, {"Operation"=enum."Clear", "Color Box"=14013909}, {"Operation"=enum."Clear", "Color Box"=14013909}, {"Operation"=enum."Clear", "Color Box"=14013909}, {"Operation"=enum."Update", "Color Box"=14013909}, {"Operation"=enum."Update", "Color Box"=16777215}, {"Operation"=enum."Clear", "Color Box"=14013909}, {"Operation"=enum."Clear", "Color Box"=14013909}, {"Operation"=enum."Clear", "Color Box"=14013909}] -> [_ _ w256 _ w280]
          tunnel: w245 -> [_ _ w255 _ w279]
          tunnel: u32[] [15790320, 15790320, 15790320, 15790320, 16777215, 16777215, 15790320, 15790320, 15790320] -> [_ _ _ _ w285]
          tunnel: w243 -> [_ _ _ _ w273]
          tunnel: w240 -> [_ w250 _ _ _]
          frame "Swerve", Default {
          }
          frame "Basic" {
            n127 = call <vilib>:"WPI_DashboardUpdateNames.vi"("Controls on Tab"=w250) -> ()  [unwired: 11 in]
          }
          frame "Test" {
            w262 = -2 ("Active Item:Row Number")
            n128 = Index Array(array=w256, index=w255) -> (element=w257:T24)
            n129 = Unbundle(w257) -> ("Operation"=w258:enum16{"Update", "Clear"}, "Color Box"=w259:u32)
            n130 = call <vilib>:"NT Read String.vi"("Name"="/TestMode/TestName") -> ("String"=w253:string)  [unwired: 9 in, 1 out]
            n131 = call <vilib>:"NT Read and Format Entries as Tree.vi"("Operation"=w258, "Name Pattern"=w263, "Tree Refnum"=w264) -> ()  [unwired: 7 in, 2 out]
            n132 = case shown="\"\"" w253 {
              tunnel: "/TestMode/TestProgress" ("Name") -> [w266 _]
              tunnel: "/TestMode/TestProgressText" ("Name") -> [w265 _]
              frame Default {
                n133 = call <vilib>:"NT Read Number.vi"("Name"=w266) -> ("Numeric"=w267:dbl)  [unwired: 9 in, 1 out]
                n134 = call <vilib>:"NT Read String.vi"("Name"=w265) -> ("String"=w268:string)  [unwired: 9 in, 1 out]
                n135 = Bundle("Numeric"=w267, "String"=w268) -> (→"Progress":cluster{"Numeric":dbl, "String":string})  [unwired: 1 in]
              }
              frame "" {
                n136 = property on="Progress" class="Clust (strict)"("Visible"=FALSE) -> ()  [unwired: 2 in, 2 out]
                n137 = local write "Test Name"(u16 0) -> ()
              }
            }
            n138 = property on="Test Tree" class="Tree (strict)"("Active Item Row Number"=w262, "ActiveColNum"=w262, "CellBG"=w259, "Active Item Row Number"=-1 ("Active Item:Row Number"), "CellBG"=u32 5789784 ("Color Box")) -> ()  [unwired: 2 in, 2 out]
          }
          frame "Variables" {
            n139 = control-ref of="Tree"() -> (w272:refnum<vi>)
            n140 = call <vilib>:"NT Read and Format Entries as Tree.vi"("Tree Refnum"=w272) -> ()  [unwired: 9 in, 2 out]
          }
          frame "Commands" {
            w281 = u32 5789784 ("Color Box")
            w282 = T25 {"Row"=-1, "Column"=-2} ("Active Cell:Active Cell")
            w284 = T25 {"Row"=-2, "Column"=-2} ("Active Cell:Active Cell")
            n141 = Index Array(array=w285, index=w279) -> (element=w283:u32)
            n142 = Index Array(array=w280, index=w279) -> (element=w278:T24)
            n143 = Unbundle(w278) -> ("Operation"=w277:enum16{"Update", "Clear"})  [unwired: 1 out]
            n144 = local read "Command Selection"() -> (w276:i32)
            n145 = property on="Command Selection" class="MCListbox (strict)"("ActiveCell"=w284, "CellBG"=w283, "ActiveCell"=w282, "CellBG"=w281) -> ()  [unwired: 2 in, 2 out]
            n146 = call <vilib>:"WPI_DashboardUpdate RPC Info.vi"("Operation"=w277) -> ("update"=w275:bool, "commands"=w274:string[][])  [unwired: 9 in]
            n147 = property on="Command Selection" class="MCListbox (strict)"("ItemNames"=w274) -> ()  [unwired: 2 in, 2 out]
            n148 = property on="Command Params" class="Tbl (strict)"("Active Cell"=w284, "Cell BG Color"=w283, "Active Cell"=w282, "Cell BG Color"=w281) -> ()  [unwired: 2 in, 2 out]
            n149 = call <vilib>:"WPI_DashboardUpdate Command Params.vi"("Update"=w275, "NewVal"=w276, "Commands"=w274, "Param Tbl"=w273) -> ()  [unwired: 7 in, 1 out]
          }
        }
        n150 = call <vilib>:"Connextion Info.vi"() -> ("Connected"=→"NT Connection":bool)  [unwired: 10 in, 1 out]
      }
      event "Test Tree": Value Change {
        # "Show appropriate\ncontrols"
        n151 = event-data() -> ("CtlRef"=w290:refnum<vi>, "NewVal"=w288:string)  [unwired: 1 in]
        n152 = call <vilib>:"WPI_UtilitiesGetTreeIOName.vi"("NewVal"=w288, "TreeControl in"=w290) -> ("I/O Name"=w291:string)  [unwired: 9 in]
        n153 = case shown="\"Camera\"" w291 {
          selector: w291 -> [_ w298 _ w320 w329 _]
          tunnel: w288 -> [_ _ w317 w319 _ w336]
          tunnel: cluster{string[]}[] [{["640x480", "320x240", "160x120"]}, {["Auto", "Fixed indoor", "Fixed outdoor 1", "Fixed outdoor 2", "Fixed fluorescent 1", "Fixed fluorescent 2", "Hold current"]}, {["Auto", "Flicker-free 50 Hz", "Flicker-free 60 Hz", "Hold current"]}, {["None", "Prioritize frame rate", "Prioritize image quality"]}, {["Monochrome", "Color"]}] -> [_ _ _ _ _ w335]
          frame Default {
            w293 = FALSE ("Visible")
            w292 = FALSE ("Visible")
            n154 = property on="Motor" class="Clust (strict)"("Visible"=w292) -> ()  [unwired: 2 in, 2 out]
            n155 = property on="Test Ring" class="Ring (strict)"("Visible"=w292) -> ()  [unwired: 2 in, 2 out]
            n156 = property on="Rev/Fwd" class="Clust (strict)"("Visible"=w293) -> ()  [unwired: 2 in, 2 out]
            n157 = property on="On/Off" class="Bool (strict)"("Visible"=w293) -> ()  [unwired: 2 in, 2 out]
            n158 = property on="Test Slider" class="Slide (strict)"("Visible"=w293) -> ()  [unwired: 2 in, 2 out]
          }
          frame "Analog Out", "Motor", "PWM" {
            w299 = FALSE ("Visible")
            n159 = case shown="\"Analog Out\"" w298 {
              tunnel: [1.0 ("Value") -1.0 ("Value") 0.0 ("Value")] -> w297
              tunnel: [255.0 ("Value") 1.0 ("Value") 5.0 ("Value")] -> w296
              tunnel: [128.0 ("Value") 0.0 ("Value") 0.0 ("Value")] -> w295
              tunnel: [64.0 ("Value") 0.5 ("Value") 1.0 ("Value")] -> w294
              frame "PWM" {
              }
              frame "Motor", Default {
              }
              frame "Analog Out" {
              }
            }
            n160 = property on="Motor" class="Clust (strict)"("Visible"=TRUE) -> ()  [unwired: 2 in, 2 out]
            n161 = property on="Value" class="Slide (strict)"("Value"=w295, "Scale.Minimum"=w297, "Scale.Maximum"=w296, "Scale.Increment"=w294) -> ()  [unwired: 2 in, 2 out]
            n162 = property on="On/Off" class="Bool (strict)"("Visible"=w299) -> ()  [unwired: 2 in, 2 out]
            n163 = property on="Test Slider" class="Slide (strict)"("Visible"=w299) -> ()  [unwired: 2 in, 2 out]
            n164 = property on="Test Ring" class="Ring (strict)"("Visible"=w299) -> ()  [unwired: 2 in, 2 out]
            n165 = property on="Rev/Fwd" class="Clust (strict)"("Visible"=w299) -> ()  [unwired: 2 in, 2 out]
          }
          frame "Servo" {
            w315 = FALSE ("Visible")
            n166 = call <vilib>:"NT Read Number.vi"("Name"=w317) -> ("Numeric"=w316:dbl)  [unwired: 9 in, 1 out]
            n167 = property on="Test Slider" class="Slide (strict)"("Visible"=TRUE, "Scale.Maximum"=170.0 ("Scale.Range:Maximum")) -> ()  [unwired: 2 in, 2 out]
            n168 = local write "Test Slider"(w316) -> ()
            n169 = property on="Motor" class="Clust (strict)"("Visible"=w315) -> ()  [unwired: 2 in, 2 out]
            n170 = property on="Rev/Fwd" class="Clust (strict)"("Visible"=w315) -> ()  [unwired: 2 in, 2 out]
            n171 = property on="On/Off" class="Bool (strict)"("Visible"=w315) -> ()  [unwired: 2 in, 2 out]
            n172 = property on="Test Ring" class="Ring (strict)"("Visible"=w315) -> ()  [unwired: 2 in, 2 out]
          }
          frame "Relay", "Solenoid" {
            w318 = FALSE ("Visible")
            n173 = property on="Motor" class="Clust (strict)"("Visible"=w318) -> ()  [unwired: 2 in, 2 out]
            n174 = property on="Test Slider" class="Slide (strict)"("Visible"=w318) -> ()  [unwired: 2 in, 2 out]
            n175 = Search and Replace String(input string=w319, search string="/Value  **", replace string="/Direction") -> (result string=w325:string)  [unwired: 5 in, 3 out]
            n176 = property on="Test Ring" class="Ring (strict)"("Visible"=w318) -> ()  [unwired: 2 in, 2 out]
            n177 = call <vilib>:"NT Read String.vi"("Name"=w325) -> ("String"=w323:string)  [unwired: 9 in, 1 out]
            n178 = Equal?(x="Both directions", y=w323) -> (x = y?=w321:bool)
            n179 = Not(x=w321) -> (.not. x?=w322:bool)
            n180 = property on="Rev/Fwd" class="Clust (strict)"("Visible"=w321) -> ()  [unwired: 2 in, 2 out]
            n181 = property on="On/Off" class="Bool (strict)"("Visible"=w322, "Caption.Text"=w320) -> ()  [unwired: 2 in, 2 out]
          }
          frame "Compressor", "Digital Out" {
            w328 = FALSE ("Visible")
            # "Get direction and finish"
            n182 = property on="Motor" class="Clust (strict)"("Visible"=w328) -> ()  [unwired: 2 in, 2 out]
            n183 = property on="Test Slider" class="Slide (strict)"("Visible"=w328) -> ()  [unwired: 2 in, 2 out]
            n184 = property on="Test Ring" class="Ring (strict)"("Visible"=w328) -> ()  [unwired: 2 in, 2 out]
            n185 = property on="On/Off" class="Bool (strict)"("Visible"=TRUE, "Caption.Text"=w329) -> ()  [unwired: 2 in, 2 out]
            n186 = property on="Rev/Fwd" class="Clust (strict)"("Visible"=FALSE) -> ()  [unwired: 2 in, 2 out]
          }
          frame "Camera" {
            n187 = call <vilib>:"Get Last Path Segment.vi"("String in"=w336) -> ("String out"=w337:string)  [unwired: 10 in]
            n188 = property on="On/Off" class="Bool (strict)"("Visible"=FALSE) -> ()  [unwired: 2 in, 2 out]
            n189 = property on="Motor" class="Clust (strict)"("Visible"=FALSE) -> ()  [unwired: 2 in, 2 out]
            n190 = property on="Rev/Fwd" class="Clust (strict)"("Visible"=FALSE) -> ()  [unwired: 2 in, 2 out]
            n191 = case shown="\"White Balance  **\"" w337 {
              tunnel: w336 -> [w343 w352 w361 w370 w379 _ w385]
              tunnel: w335 -> [w341 w349 w358 w367 w376 _ _]
              frame "Size  **" {
                n192 = Index Array(array=w341) -> (element=w340:cluster{string[]})  [unwired: 1 in]
                n193 = call <vilib>:"NT Read String.vi"("Name"=w343) -> ("String"=w342:string)  [unwired: 9 in, 1 out]
                n194 = Unbundle(w340) -> (w338:string[])
                n195 = Match First String(2:w338, 3:w342) -> (0:w339:i32)  [unwired: 1 out]
                n196 = property on="Test Ring" class="Ring (strict)"("Value"=w339, "Strings []"=w338) -> ()  [unwired: 2 in, 2 out]
                n197 = property on="Test Ring" class="Ring (strict)"("Visible"=TRUE) -> ()  [unwired: 2 in, 2 out]
                n198 = property on="Test Slider" class="Slide (strict)"("Visible"=FALSE) -> ()  [unwired: 2 in, 2 out]
              }
              frame "White Balance  **" {
                n199 = Index Array(array=w349, index=1) -> (element=w350:cluster{string[]})
                n200 = call <vilib>:"NT Read String.vi"("Name"=w352) -> ("String"=w351:string)  [unwired: 9 in, 1 out]
                n201 = Unbundle(w350) -> (w347:string[])
                n202 = Match First String(2:w347, 3:w351) -> (0:w346:i32)  [unwired: 1 out]
                n203 = property on="Test Ring" class="Ring (strict)"("Value"=w346, "Strings []"=w347) -> ()  [unwired: 2 in, 2 out]
                n204 = property on="Test Ring" class="Ring (strict)"("Visible"=TRUE) -> ()  [unwired: 2 in, 2 out]
                n205 = property on="Test Slider" class="Slide (strict)"("Visible"=FALSE) -> ()  [unwired: 2 in, 2 out]
              }
              frame "Exposure  **" {
                n206 = Index Array(array=w358, index=2) -> (element=w359:cluster{string[]})
                n207 = call <vilib>:"NT Read String.vi"("Name"=w361) -> ("String"=w360:string)  [unwired: 9 in, 1 out]
                n208 = Unbundle(w359) -> (w355:string[])
                n209 = Match First String(2:w355, 3:w360) -> (0:w356:i32)  [unwired: 1 out]
                n210 = property on="Test Ring" class="Ring (strict)"("Value"=w356, "Strings []"=w355) -> ()  [unwired: 2 in, 2 out]
                n211 = property on="Test Ring" class="Ring (strict)"("Visible"=TRUE) -> ()  [unwired: 2 in, 2 out]
                n212 = property on="Test Slider" class="Slide (strict)"("Visible"=FALSE) -> ()  [unwired: 2 in, 2 out]
              }
              frame "Exposure Priority  **" {
                n213 = Index Array(array=w367, index=3) -> (element=w368:cluster{string[]})
                n214 = call <vilib>:"NT Read String.vi"("Name"=w370) -> ("String"=w369:string)  [unwired: 9 in, 1 out]
                n215 = Unbundle(w368) -> (w364:string[])
                n216 = Match First String(2:w364, 3:w369) -> (0:w365:i32)  [unwired: 1 out]
                n217 = property on="Test Ring" class="Ring (strict)"("Value"=w365, "Strings []"=w364) -> ()  [unwired: 2 in, 2 out]
                n218 = property on="Test Ring" class="Ring (strict)"("Visible"=TRUE) -> ()  [unwired: 2 in, 2 out]
                n219 = property on="Test Slider" class="Slide (strict)"("Visible"=FALSE) -> ()  [unwired: 2 in, 2 out]
              }
              frame "Color Enable  **" {
                n220 = Index Array(array=w376, index=4) -> (element=w377:cluster{string[]})
                n221 = call <vilib>:"NT Read String.vi"("Name"=w379) -> ("String"=w378:string)  [unwired: 9 in, 1 out]
                n222 = Unbundle(w377) -> (w373:string[])
                n223 = Match First String(2:w373, 3:w378) -> (0:w374:i32)  [unwired: 1 out]
                n224 = property on="Test Ring" class="Ring (strict)"("Value"=w374, "Strings []"=w373) -> ()  [unwired: 2 in, 2 out]
                n225 = property on="Test Ring" class="Ring (strict)"("Visible"=TRUE) -> ()  [unwired: 2 in, 2 out]
                n226 = property on="Test Slider" class="Slide (strict)"("Visible"=FALSE) -> ()  [unwired: 2 in, 2 out]
              }
              frame Default {
                n227 = property on="Test Ring" class="Ring (strict)"("Visible"=FALSE) -> ()  [unwired: 2 in, 2 out]
                n228 = property on="Test Slider" class="Slide (strict)"("Visible"=FALSE) -> ()  [unwired: 2 in, 2 out]
              }
              frame "Brightness  **", "Color Level  **", "Compression  **", "FPS  **", "Sharpness  **" {
                n229 = call <vilib>:"NT Read Number.vi"("Name"=w385) -> ("Numeric"=w384:dbl)  [unwired: 9 in, 1 out]
                n230 = local write "Test Slider"(w384) -> ()
                n231 = property on="Test Slider" class="Slide (strict)"("Visible"=TRUE, "Scale.Maximum"=100.0 ("Scale.Range:Maximum")) -> ()  [unwired: 2 in, 2 out]
                n232 = property on="Test Ring" class="Ring (strict)"("Visible"=FALSE) -> ()  [unwired: 2 in, 2 out]
              }
            }
          }
        }
        n233 = property on="Progress" class="Clust (strict)"("Visible"=FALSE) -> ()  [unwired: 2 in, 2 out]
      }
      event "Test Name": Mouse Enter {
        # "Populate the ring with the list of tests"
        n234 = event-data() -> ()  [unwired: 1 in, 1 out]
        n235 = call <vilib>:"NT Read String Array.vi"("Name"="/TestMode/TestList") -> ("String Array"=w393:string[])  [unwired: 9 in, 1 out]
        n236 = Build Array (concatenate)("Select the test to run...", w393) -> (w392:string[])
        n237 = property on="Test Name" class="Ring (strict)"("Strings []"=w392) -> ()  [unwired: 2 in, 2 out]
      }
      event "Test Name": Value Change {
        w395 = FALSE ("Visible")
        # "Tell the robot the test name to run"
        n238 = event-data() -> ("NewVal"=w399:u16)  [unwired: 1 in]
        n239 = property on="Test Name" class="Ring (strict)"() -> ("Strings []"=w400:string[])  [unwired: 2 in, 2 out]
        n240 = local write "Progress"(T7 {"Test Progress"=0, "Test Progress Text"=""} ("Progress")) -> ()
        n241 = Index Array(array=w400, index=w399) -> (element=w398:string)
        n242 = call <vilib>:"NT Write String.vi"("String"=w398, "Name"="/TestMode/TestName") -> ()  [unwired: 9 in, 1 out]
        n243 = property on="Progress" class="Clust (strict)"("Visible"=TRUE) -> ()  [unwired: 2 in, 2 out]
        n244 = property on="Motor" class="Clust (strict)"("Visible"=w395) -> ()  [unwired: 2 in, 2 out]
        n245 = property on="Test Slider" class="Slide (strict)"("Visible"=w395) -> ()  [unwired: 2 in, 2 out]
        n246 = property on="On/Off" class="Bool (strict)"("Visible"=w395) -> ()  [unwired: 2 in, 2 out]
        n247 = property on="Rev/Fwd" class="Clust (strict)"("Visible"=w395) -> ()  [unwired: 2 in, 2 out]
        n248 = property on="Test Ring" class="Ring (strict)"("Visible"=w395) -> ()  [unwired: 2 in, 2 out]
      }
      event "Select Auto": Mouse Enter {
        # "Populate the combo box with the list of autonomous options"
        n249 = event-data() -> ()  [unwired: 1 in, 1 out]
        n250 = call <vilib>:"NT Read String Array.vi"("Name"="Auto List") -> ("String Array"=w402:string[])  [unwired: 9 in, 1 out]
        n251 = property on="Select Auto" class="CmbBox"("Strings[]"=w402) -> ()  [unwired: 2 in, 2 out]
      }
      event "Select Auto": Value Change {
        # "User modified the Auto Selection. Write to NT variable so robot knows."
        n252 = event-data() -> ("NewVal"=w405:string)  [unwired: 1 in]
        n253 = call <vilib>:"NT Write String.vi"("String"=w405, "Name"="Auto Selector") -> ()  [unwired: 9 in, 1 out]
      }
      event "Command Selection": Value Change {
        # "Get the params and show in table"
        n254 = event-data() -> ("NewVal"=w411:i32)  [unwired: 1 in]
        n255 = property on="Command Selection" class="MCListbox (strict)"() -> ("ItemNames"=w409:string[][])  [unwired: 2 in, 2 out]
        n256 = call <vilib>:"WPI_DashboardUpdate Command Params.vi"("NewVal"=w411, "Commands"=w409, "Param Tbl"=w410) -> ()  [unwired: 8 in, 1 out]
      }
      event "Execute Command": Value Change {
        # "Started one, Unique ID holds\nresponse"
        n257 = event-data() -> ()  [unwired: 1 in, 1 out]
        n258 = property on="Command Selection" class="MCListbox (strict)"() -> ("ItemNames"=w422:string[][])  [unwired: 2 in, 2 out]
        n259 = Index Array(array=w422, index (row)="Command Selection", index (col)=0) -> (element=w420:string)
        n260 = call <vilib>:"Invoke Commands.vi"("Command Params"="Command Params", "Function Name"=w420) -> ("Params"=w416:u8, "Started"=w415:bool)  [unwired: 7 in, 1 out]
        n261 = Array Subset(array="Command Params", length (row)=w416) -> (w417:string[][])  [unwired: 3 in]
        n262 = Select(t="Executing" ("Cmd Status"), s=w415, f="" ("Cmd Status")) -> (s? t:f=→"Cmd Status":string)
      }
      event "Command Selection": Double Click {
        n263 = event-data() -> ("Row"=w430:i32)  [unwired: 1 in]
        n264 = property on="Command Selection" class="MCListbox (strict)"() -> ("ItemNames"=w433:string[][])  [unwired: 2 in, 2 out]
        n265 = local read "Command Params"() -> (w429:string[][])
        n266 = Index Array(array=w433, index (row)=w430, index (col)=0) -> (element=w431:string)
        n267 = call <vilib>:"Invoke Commands.vi"("Command Params"=w429, "Function Name"=w431) -> ("Params"=w428:u8, "Started"=w423:bool)  [unwired: 7 in, 1 out]
        n268 = Array Subset(array=w429, length (row)=w428) -> (w427:string[][])  [unwired: 3 in]
        n269 = Select(t="Executing" ("Cmd Status"), s=w423, f="" ("Cmd Status")) -> (s? t:f=w424:string)
        n270 = local write "Cmd Status"(w424) -> ()
      }
      event "CheckList": Double Click {
        # "Shift clears all"
        # "Update symbols on the listbox"
        n271 = event-data() -> ("PlatMods.Shift"=w435:bool, "Row"=w437:i32)  [unwired: 1 in]
        n272 = case shown="True" w435 {
          tunnel: w437 -> [w441 _]
          tunnel: 1 -> [w440 _]
          frame False {
            n273 = property on="CheckList" class="LstBox (strict)"() -> ("Item Symbols"=w439:i32[])  [unwired: 2 in, 2 out]
            n274 = Replace Array Subset(array=w439, new element=w440, index=w441) -> (w438:i32[])
            n275 = property on="CheckList" class="LstBox (strict)"("Item Symbols"=w438) -> ()  [unwired: 2 in, 2 out]
          }
          frame True {
            w442 = 0 ("Top Row")
            n276 = property on="CheckList" class="LstBox (strict)"() -> ("Number of Rows"=w444:u32)  [unwired: 2 in, 2 out]
            n277 = Initialize Array(0, w444) -> (w443:i32[])
            n278 = property on="CheckList" class="LstBox (strict)"("Top Row"=w442, "Value"=w442, "Item Symbols"=w443) -> ()  [unwired: 2 in, 2 out]
          }
        }
      }
      event "CheckList": Key Down {
        # "Update symbols on the listbox\nLeft and right keys check and uncheck"
        n279 = event-data() -> ("VKey"=w448:T22)  [unwired: 1 in]
        n280 = case shown="\"Left\", \"Right\"" w448 {
          selector: w448 -> [w453 _]
          tunnel: eventvkey."Left" ("VKey") -> [w451 _]
          frame "Left", "Right" {
            n281 = Equal?(x=w451, y=w453) -> (x = y?=w452:bool)
            n282 = Select(t=0, s=w452, f=1) -> (s? t:f=w454:i32)
            n283 = property on="CheckList" class="LstBox (strict)"() -> ("Item Symbols"=w457:i32[])  [unwired: 2 in, 2 out]
            n284 = Replace Array Subset(array=w457, new element=w454, index="CheckList") -> (w456:i32[])
            n285 = property on="CheckList" class="LstBox (strict)"("Item Symbols"=w456) -> ()  [unwired: 2 in, 2 out]
          }
          frame Default {
          }
        }
      }
      event "Motor.Enable": Value Change {
        # "When the test mode otor enable helper is set, update that\ntree row item's value"
        n286 = event-data() -> ("NewVal"=w463:bool)  [unwired: 1 in]
        n287 = Unbundle("Motor") -> ("Value"=w462:dbl)  [unwired: 1 out]
        n288 = Select(t=w462, s=w463, f=0.0) -> (s? t:f=w460:dbl)
        n289 = call <vilib>:"NT Write Number.vi"("Numeric"=w460, "Name"=w459) -> ()  [unwired: 9 in, 1 out]
      }
      event "Test Slider": Value Change {
        # "When the test mode slider helper is set, update that\ntree row item's value"
        n290 = event-data() -> ("NewVal"=w466:dbl)  [unwired: 1 in]
        n291 = call <vilib>:"NT Write Number.vi"("Numeric"=w466, "Name"=w467) -> ()  [unwired: 9 in, 1 out]
      }
      event "On/Off": Value Change {
        # "When the test mode on/off helper value is set, update that\ntree row item's value"
        n292 = event-data() -> ("NewVal"=w471:bool)  [unwired: 1 in]
        n293 = Boolean To (0,1)(Boolean=w471) -> (0, 1=w470:i16)
        n294 = call <vilib>:"NT Write Number.vi"("Numeric"=w470, "Name"=w469) -> ()  [unwired: 9 in, 1 out]
      }
      event "Rev/Fwd": Value Change {
        # "When the test mode helper value for relays is set, update that\ntree row item's value"
        n295 = event-data() -> ("NewVal.Forward"=w479:bool, "NewVal.Reverse"=w478:bool)  [unwired: 1 in]
        n296 = Boolean To (0,1)(Boolean=w479) -> (0, 1=w475:i16)
        n297 = Boolean To (0,1)(Boolean=w478) -> (0, 1=w477:i16)
        n298 = Negate(x=w477) -> (-x=w476:i16)
        n299 = Add(x=w475, y=w476) -> (x+y=w474:i16)
        n300 = call <vilib>:"NT Write Number.vi"("Numeric"=w474, "Name"=w473) -> ()  [unwired: 9 in, 1 out]
      }
      event "Test Ring": Value Change {
        # "When a test mode helper value is selected from the ring,\nset the tree item's variable to the string value"
        n301 = event-data() -> ("NewVal"=w483:u16)  [unwired: 1 in]
        n302 = property on="Test Ring" class="Ring (strict)"() -> ("Strings []"=w484:string[])  [unwired: 2 in, 2 out]
        n303 = Index Array(array=w484, index=w483) -> (element=w482:string)
        n304 = call <vilib>:"NT Write String.vi"("String"=w482, "Name"=w481) -> ()  [unwired: 9 in, 1 out]
      }
      event "Rec Mode": Value Change {
        # "Update globals for recording mode and path to read log from.\nClear when logging and let NetworkTables set path for vision to\nuse."
        n305 = event-data() -> ("NewVal"=w495:enum32{"Stop", "Record", "Playback"})  [unwired: 1 in]
        n306 = global write "WPI_DashboardLogging Global.vi" "Logging Filename"(path "") -> ()
        n307 = global write "WPI_DashboardLogging Global.vi" "Recording"(w495) -> ()
        n308 = case shown="\"Playback\"" w495 {
          tunnel: w494 -> [_ w497 w506]
          tunnel: [_ _ w505] -> w492
          tunnel: [_ _ w504] -> _
          tunnel: w490 -> [_ _ w502]
          tunnel: cluster{i32, i32} {-250, 170} -> [_ _ w501]
          tunnel: [_ _ T23 {"Image Size"=TRUE, "Image Type"=TRUE, "Pixel Value"=TRUE, "ROI Information"=TRUE, "Zoom Factor"=FALSE} ("Image Information Shown:All Elements")] -> w488
          tunnel: [_ _ TRUE ("Zoom Factor")] -> w487
          tunnel: w486 -> [_ _ w498]
          frame Default {
          }
          frame "Stop", "Record" {
            # "Place Window too"
            n309 = invoke class="VI" method="FP.Close"(reference=w497) -> (reference out=w496:refnum<vi>)  [unwired: 2 in, 2 out]
            n310 = invoke class="VI" method="Abort VI"(reference=w496) -> ()  [unwired: 2 in, 3 out]
          }
          frame "Playback" {
            n311 = call "Open Playback Panel.vi"("Offset"=w501, "DB VI Ref"=w502, "Playback in"=w506) -> ("Playback out"=w503:refnum<vi>)  [unwired: 8 in]
            n312 = register-events(w503, w498) -> (reference out=w505:refnum<event-registration>, error out=w504:errorcluster)  [unwired: 2 in]
          }
        }
        n313 = property on="Camera Image" class="ImageControl"("Image Information Shown"=w488, "Image Information Visible"=w487) -> ()  [unwired: 2 in, 2 out]
        n314 = call <vilib>:"WPI_DashboardNT Log FieldName Cache.vi"("Operation"=enum16{"Lookup/Add", "Index", "Clear"}."Clear") -> ()  [unwired: 8 in, 3 out]
      }
      event Panel Close {
        w508 = enum32{"Stop", "Record", "Playback"}."Stop" ("Rec Mode")
        # "Playback window has been closed, abort"
        n315 = event-data() -> ()  [unwired: 1 in, 4 out]
        n316 = local write "Rec Mode"(w508) -> ()
        n317 = global write "WPI_DashboardLogging Global.vi" "Recording"(w508) -> ()
      }
      event Panel Close {
        # "Abort playback window and ourself"
        n318 = event-data() -> ()  [unwired: 1 in, 4 out]
        n319 = invoke class="VI" method="FP.Close"(reference=w512) -> (reference out=w511:refnum<vi>)  [unwired: 2 in, 2 out]
        n320 = invoke class="VI" method="Abort VI"(reference=w511) -> (error out=w510:errorcluster)  [unwired: 2 in, 2 out]
        n321 = invoke class="VI" method="Abort VI"(error in=w510) -> ()  [unwired: 2 in, 3 out]
      }
      event User Event {
        n322 = event-data() -> ("IDs"=w519:cluster{"RPC field ID":u16, "Unique ID":u16}, "String"=w518:string)  [unwired: 1 in]
        n323 = Bundle("IDs"=w519, "String"=w518) -> (w517:T9)  [unwired: 1 in]
        n324 = call <vilib>:"Retrieve RPC Response.vi"("RPC Response"=w517) -> ("Output"=w515:string[][])  [unwired: 10 in]
        n325 = Build Array (concatenate)(w513, w515) -> (w514:string[][])
        n326 = local write "Command Params"(w514) -> ()
        n327 = local write "Cmd Status"("" ("Cmd Status")) -> ()
      }
      event "Tree": Double Click {
        n328 = event-data() -> ("PlatMods"=w523:T26, "Tag"=w522:string)  [unwired: 1 in]
        n329 = Unbundle(w523) -> ("Shift"=w521:bool)  [unwired: 4 out]
        n330 = Not(x=w521) -> (.not. x?=w520:bool)
        n331 = call <vilib>:"NT Update Persistence.vi"("Persistence"=w520, "Name"=w522) -> ()  [unwired: 9 in, 1 out]
      }
    }
  }
  n332 = while {
    tunnel: w64 -> [w526]
    i -> [w529]
    stop <- FALSE stop-if-true
    n333 = Wait (ms)(milliseconds to wait=u32 100) -> ()  [unwired: 1 out]
    n334 = case shown="\"Playback\"" "Rec Mode" {
      tunnel: w529 -> [_ _ w544]
      tunnel: [u32 2829099 ("Base Color") u32 11141120 ("Target Color") w533] -> w525
      frame "Stop", Default {
        # "Reset the color, extra updates don't cost much"
      }
      frame "Record" {
      }
      frame "Playback" {
        # "Playback"
        n335 = Quotient & Remainder(x=w544, y=u32 50 ("milliseconds to wait")) -> (x-y*floor(x/y)=w540:u32)  [unwired: 1 out]
        n336 = Divide(x=w540, y=u32 50 ("milliseconds to wait")) -> (x/y=w537:dbl)
        n337 = Multiply(x=6.283185307179586, y=w537) -> (x*y=w542:dbl)
        n338 = Sine(x=w542) -> (sin(x)=w541:dbl)
        n339 = Absolute Value(x=w541) -> (abs(x)=w534:dbl)
        n340 = call "Interpolate RGB Color.vi"("Proportion"=w534, "Target Color"=u32 30976, "Base Color"=u32 2829099) -> ("Result Color"=w533:u32)  [unwired: 8 in]
      }
    }
    n341 = property class="Pane"(reference=w526, "PaneColor"=w525) -> ()  [unwired: 1 in, 2 out]
  }
  n342 = local write "Dashboard Tab"(T2."Swerve" ("Dashboard Tab")) -> ()
  n343 = property on="On/Off" class="Bool (strict)"("Visible"=w33) -> ()  [unwired: 2 in, 2 out]
  n344 = property on="Motor" class="Clust (strict)"("Visible"=w33) -> ()  [unwired: 2 in, 2 out]
  n345 = property on="Progress" class="Clust (strict)"("Visible"=w33) -> ()  [unwired: 2 in, 2 out]
  n346 = property on="Test Ring" class="Ring (strict)"("Visible"=w33) -> ()  [unwired: 2 in, 2 out]
  n347 = property on="Rev/Fwd" class="Clust (strict)"("Visible"=w33) -> ()  [unwired: 2 in, 2 out]
  n348 = while {
    tunnel: u16 1741 ("timeout ms (25000)") -> [w546]
    stop <- FALSE stop-if-true
    n349 = TCP Create Listener(10:w546) -> (0:w545:errorcluster, 3:w547:refnum<k5>)  [unwired: 4 in, 1 out]
    n350 = case shown="No Error" w545 {
      selector: w545 -> [w549 _]
      tunnel: w547 -> [w550 _]
      frame No Error {
        n351 = while {
          tunnel: w550 -> [w553]
          tunnel: w549 -> [w552]
          stop <- FALSE stop-if-true
          n352 = TCP Wait On Listener(8:w552, 11:w553) -> (0:w554:errorcluster, 4:w555:refnum<k5>)  [unwired: 2 in, 3 out]
          n353 = local write "TCP"(w555) -> ()
          n354 = case shown="No Error" w554 {
            frame No Error {
            }
            frame Error {
              n355 = Wait (ms)(milliseconds to wait=u32 1000) -> ()  [unwired: 1 out]
            }
          }
        }
      }
      frame Error {
        n356 = Wait (ms)(milliseconds to wait=u32 1000) -> ()  [unwired: 1 out]
      }
    }
  }
  n357 = local write "Command Selection"(u16 0 ("milliseconds to wait")) -> ()
  n358 = local write "Command Params"(string[][] [] ("Command Params")) -> ()
  n359 = global write "WPI_DashboardLogging Global.vi" "Recording"(w58) -> ()
  n360 = local write "Rec Mode"(w58) -> ()
  n361 = call <vilib>:"NT Write String.vi"("String"="Select Auto", "Name"="Auto Selector") -> ()  [unwired: 9 in, 1 out]
